vi "VHMI-recieveStatus.vi"(8 "error in (no error)":errorcluster, 11 "VHMI-VNA_Hardware_manager_Interface in":refnum<class "VHMI-VNA_Hardware_manager_Interface.lvclass">) -> (0 "error out":errorcluster, 3 "VHMI-VNA_Hardware_manager_Interface out":refnum<class "VHMI-VNA_Hardware_manager_Interface.lvclass">)   [LabVIEW 2020, in "VHMI-VNA_Hardware_manager_Interface.lvlib" / "VHMI-VNA_Hardware_manager_Interface.lvclass"]
uses:
  VHMI-VNA_Hardware_manager_Interface.lvclass
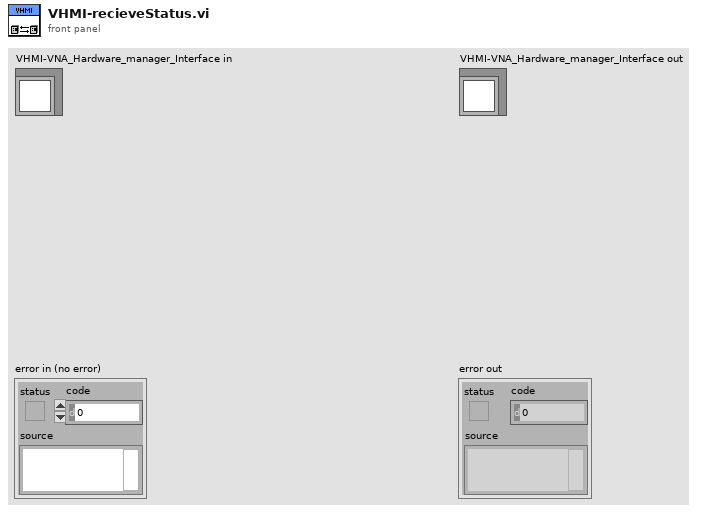
[diagram p1: front panel]
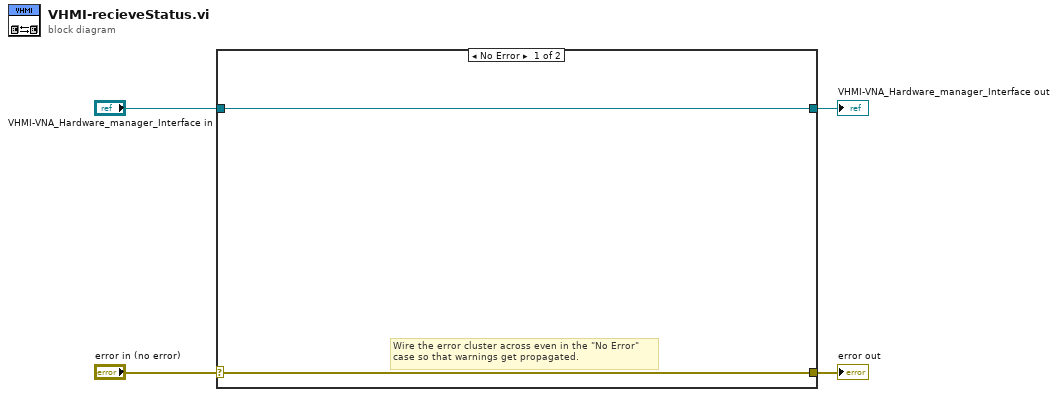
[diagram p0: block diagram]
diagram:
  n1 = case shown="No Error" "error in (no error)" {
    selector: "error in (no error)" -> [w5 w8]
    tunnel: [w5 w8] -> w3
    tunnel: [w6 w7] -> w1
    tunnel: "VHMI-VNA_Hardware_manager_Interface in" -> [w6 w7]
    frame No Error {
      # "Wire the error cluster across even in the \"No Error\"\ncase so that warnings get propagated."
    }
    frame Error {
    }
  }
  "error out" <- w3
  "VHMI-VNA_Hardware_manager_Interface out" <- w1
